vi "Get text file line count.vi"(8 "error in (no error)":errorcluster, 10 "Text file":path, 11 "text string":string) -> (0 "error out":errorcluster, 3 "Line cnt":i32)   [LabVIEW 2013]
doc: "To get the last line counted, you must have a carriage return or linefeed\nIf text file input isn't empty, then a file will be read instead of text input box"
panel:
  out "LF cnt":i32
  out "CR cnt":i32
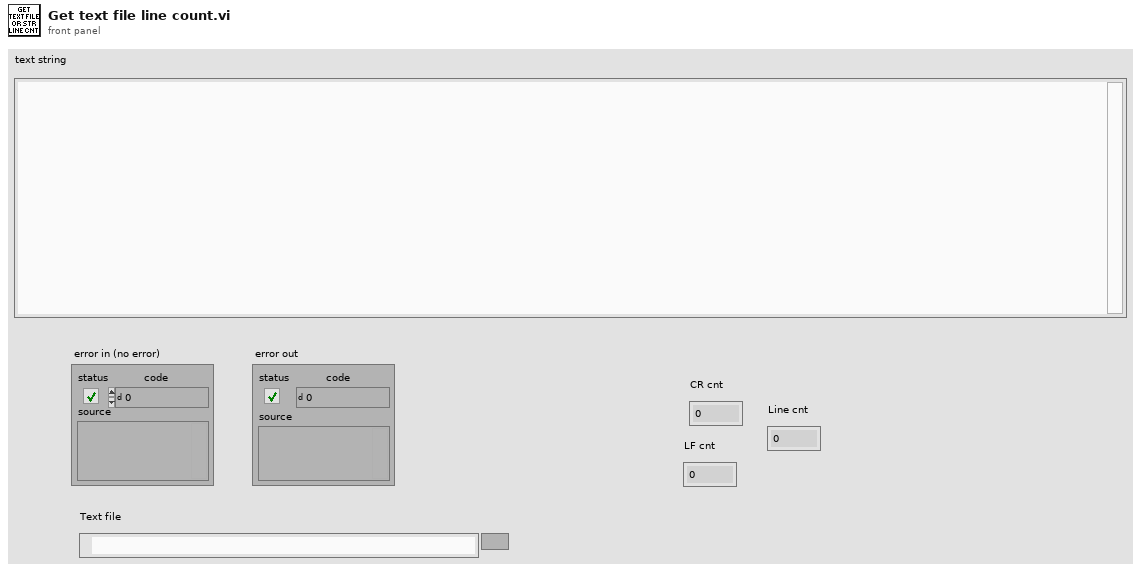
[diagram p1: front panel]
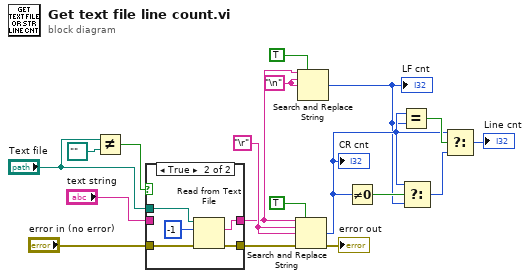
[diagram p0: block diagram]
diagram:
  w14 = "\n"
  w18 = "\r"
  n1 = Not Equal?(x="Text file", y=path "") -> (x != y?=w5:bool)
  n2 = case shown="True" w5 {
    tunnel: "Text file" -> [_ w25]
    tunnel: "text string" -> [w19 _]
    tunnel: "error in (no error)" -> [w20 w24]
    tunnel: [w20 w23] -> w2
    tunnel: [w19 w22] -> w1
    frame False {
    }
    frame True {
      n3 = Read from Text File(file (use dialog)=w25, count=-1, error in=w24) -> (text=w22:string, error out=w23:errorcluster)  [unwired: 1 in, 2 out]
    }
  }
  n4 = Search and Replace String(replace all?=TRUE ("replace all? (F)"), input string=w1, search string=w18, replace string=w18, error in=w2) -> (number of replacements=w10:i32, error out=→"error out":errorcluster)  [unwired: 3 in, 2 out]
  "CR cnt" <- w10
  n5 = Search and Replace String(replace all?=TRUE ("replace all? (F)"), input string=w1, search string=w14, replace string=w14) -> (number of replacements=w9:i32)  [unwired: 4 in, 3 out]
  "LF cnt" <- w9
  n6 = Not Equal To 0?(x=w10) -> (x != 0?=w11:bool)
  n7 = Equal?(x=w10, y=w9) -> (x = y?=w13:bool)
  n8 = Select(t=w10, s=w11, f=w9) -> (s? t:f=w8:i32)
  n9 = Select(t=w10, s=w13, f=w8) -> (s? t:f=→"Line cnt":i32)
